vi "getStatus.vi"(0 "reference (in)":refnum<class "_SingleAxisController.lvclass">, 2 "nc (single axis controllers require no axis specification)":T5, 5 "error in (no error)":errorcluster) -> (14 "reference (out)":refnum<class "_SingleAxisController.lvclass">, 16 "status (raw result)":string, 17 "full_state":T1={"X"={"motion_state"=enum."CONST", "other_states"=[]}, "Y"={"motion_state"=enum."CONST", "other_states"=[]}, "Z"={"motion_state"=enum."CONST", "other_states"=[]}, "U"={"motion_state"=enum."CONST", "other_states"=[]}, "buffer_enabled?"=FALSE, "buffer_start"=0, "buffer_end"=0, "avail_buffer"=0, "move_mode"=enum."ABSOLUTE"}, 19 "error out":errorcluster)   [LabVIEW 2013, in "classes.lvlib" / "_SingleAxisController.lvclass"]
doc: "Produced By:\n\n<B>Kod Integrations, LLC</B>\n4835 Marianne Drive\nMount Airy, MD 21771\nhttp://www.kodintegrations.com\nemail: info@kodintegrations.com\nphone: (240) 687-1288"
uses:
  _SingleAxisController.lvclass
  axis.ctl
  complete_motor_state.ctl
  single_axis_state.ctl
  motor_status.ctl
  move_mode.ctl
  _Controller.lvclass
  common.lvlib
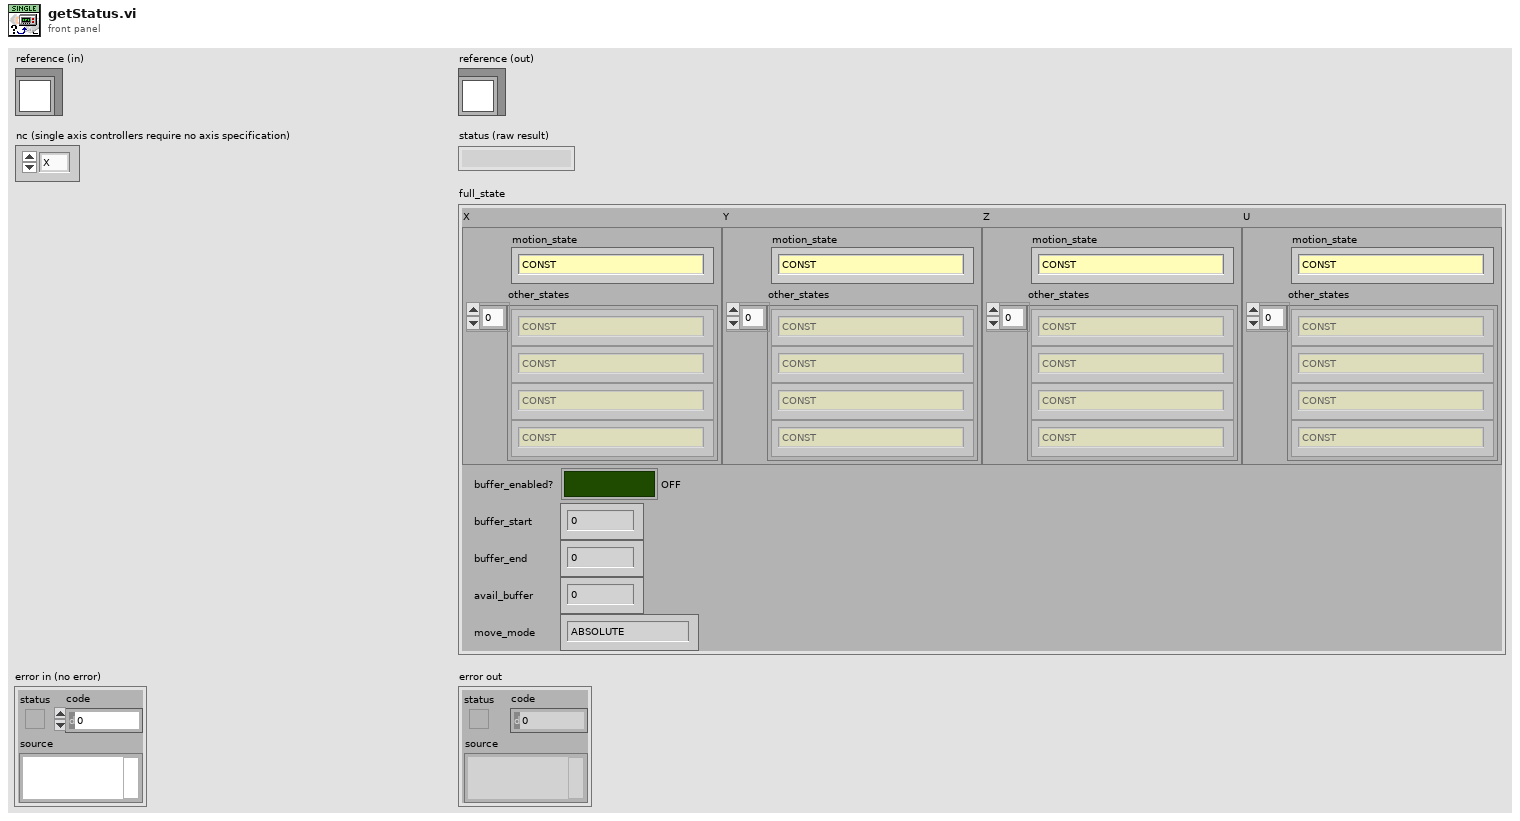
[diagram p1: front panel]
types:
  T1 = typedef "common.lvlib/complete_motor_state.ctl" = cluster{"X":T2, "Y":T2, "Z":T2, "U":T2, "buffer_enabled?":bool, "buffer_start":i32, "buffer_end":i32, "avail_buffer":i32, "move_mode":T4}
  T2 = typedef "common.lvlib/single_axis_state.ctl" = cluster{"motion_state":T3, "other_states":T3[]}
  T3 = typedef "common.lvlib/motor_status.ctl" = enum16{"IDLE", "CONST", "ACCEL", "DECEL", "HOME_SWITCH", "-LIMIT_SWITCH", "+LIMIT_SWITCH", "-LIMIT_ERR", "+LIMIT_ERR", "COMM_TIMEOUT", "ALARM_INPUT", "ALARM_ERROR", "TOC_TIMEOUT_STATUS", "LATCH_INPUT_STATUS", "Z_INDEX_STATUS"}
  T4 = typedef "common.lvlib/move_mode.ctl" = enum16{"ABSOLUTE", "INCREMENTAL"}
  T5 = typedef "common.lvlib/axis.ctl" = enum16{"X", "Y", "Z", "U"}
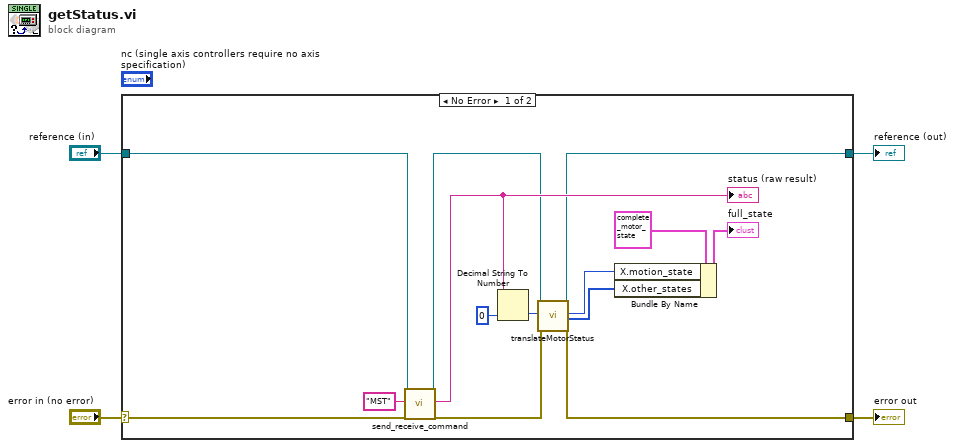
[diagram p0: block diagram]
diagram:
  n1 = case shown="No Error" "error in (no error)" {
    selector: "error in (no error)" -> [w16 w20]
    tunnel: [w5 w20] -> w3
    tunnel: [w11 w19] -> w1
    tunnel: "reference (in)" -> [w14 w19]
    frame No Error {
      n2 = call "send_receive_command.vi"("reference (in)"=w14, "ASCII Command (in)"="MST", "error in (no error)"=w16) -> ("reference (out)"=w12:refnum<class "_SingleAxisController.lvclass">, "response (out)"=w13:string, "error out"=w6:errorcluster)  [unwired: 12 in, 2 out]
      "status (raw result)" <- w13
      n3 = Decimal String To Number(string=w13, default (0L)=u32 0 ("default (0 I32)")) -> (number=w17:u32)  [unwired: 1 in, 1 out]
      n4 = call-dynamic "translateMotorStatus.vi"("Controller in"=w12, "actual value"=w17, "error in (no error)"=w6) -> ("Controller out"=w11:refnum<class "_SingleAxisController.lvclass">, "motion_state"=w8:T3, "other_states (for use in overiding classes)"=w7:T3[], "error out"=w5:errorcluster)  [unwired: 13 in]
      n5 = Bundle By Name(cluster=T1 {"X"={"motion_state"=enum."IDLE", "other_states"=[]}, "Y"={"motion_state"=enum."IDLE", "other_states"=[]}, "Z"={"motion_state"=enum."IDLE", "other_states"=[]}, "U"={"motion_state"=enum."IDLE", "other_states"=[]}, "buffer_enabled?"=FALSE, "buffer_start"=0, "buffer_end"=0, "avail_buffer"=0, "move_mode"=enum."INCREMENTAL"} ("full_state"), "X.motion_state"=w8, "X.other_states"=w7) -> (→"full_state":T1)
    }
    frame Error {
    }
  }
  "error out" <- w3
  "reference (out)" <- w1
